vi "getImage.vi"(4 "Streeam":bool, 5 "imageError IN":errorcluster, 6 "Image IN":T1, 7 "errorCamera IN":errorcluster, 8 "hCamera IN":u32) -> (0 "errorImage OUT":errorcluster, 1 "Image OUT":T1, 2 "errorCamera OUT":errorcluster, 3 "hCamera OUT":u32)   [LabVIEW 2010]
uses:
  <vilib>/vision/Image Controls.llb/IMAQ Image.ctl
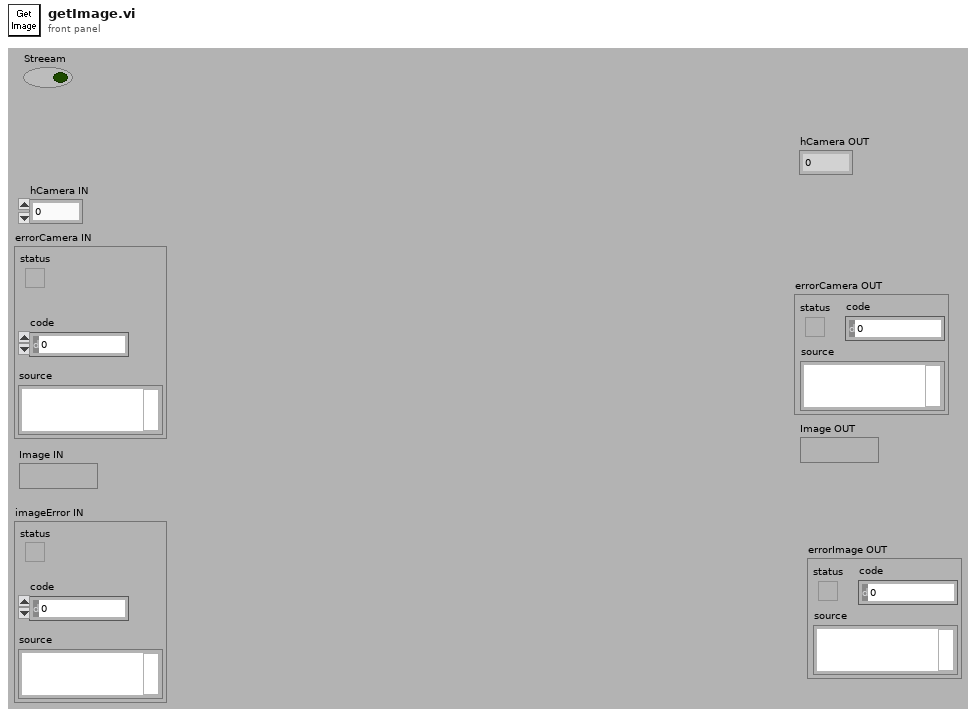
[diagram p1: front panel]
types:
  T1 = typedef "IMAQ Image.ctl" = refnum<image>
  T2 = enum32{"Map Pixel Pointer", "Unmap Pixel Pointer", "Get Pixels Infos"}
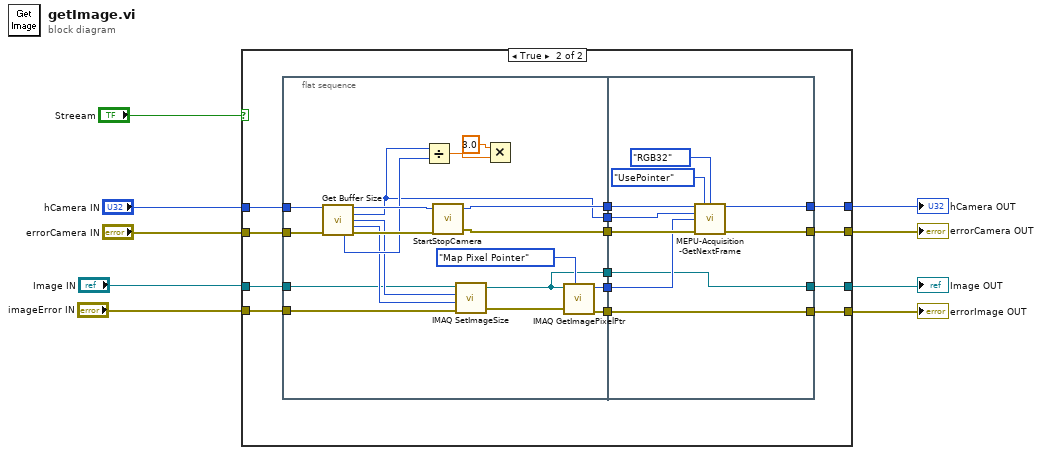
[diagram p0: block diagram]
diagram:
  n1 = case shown="True" "Streeam" {
    tunnel: "hCamera IN" -> [w13 w22]
    tunnel: "errorCamera IN" -> [w12 w21]
    tunnel: "Image IN" -> [w11 w20]
    tunnel: "imageError IN" -> [w10 w19]
    tunnel: [w11 w18] -> w4
    tunnel: [w10 w17] -> w3
    tunnel: [w12 w16] -> w2
    tunnel: [w13 w15] -> w1
    frame False {
    }
    frame True {
      n2 = flat-sequence {
        tunnel: [w44] -> w27
        tunnel: [w43] -> w26
        tunnel: w20 -> [w37]
        tunnel: w19 -> [w36]
        tunnel: w22 -> [w35]
        tunnel: w21 -> [w34]
        tunnel: [w31] -> w25
        tunnel: [w30] -> w24
        tunnel: [w29] -> w23
        tunnel: [w28] -> w14
        tunnel: w27 -> [w56]
        tunnel: w26 -> [w55]
        tunnel: w25 -> [w51]
        tunnel: w24 -> [w48]
        tunnel: w23 -> [w49]
        tunnel: [w50] -> w15
        tunnel: [w49] -> w18
        tunnel: [w48] -> w17
        tunnel: [w47] -> w16
        tunnel: w14 -> [w54]
        frame #0 {
          n3 = call "Get Buffer Size.vi"("phCamera IN"=w35, "Error IN"=w34) -> ("phCamera OUT"=w46:u32, "uBufferSize OUT"=w28:u32, "uWidth OUT"=w39:u32, "uHeight OUT"=w38:u32, "uBytesPerPixel OUT"=w40:u32, "Error OUT"=w45:errorcluster)  [unwired: 8 out]
          n4 = Divide(x=w28, y=w40) -> (x/y=w42:dbl)
          n5 = call "StartStopCamera.vi"("Error IN"=w45, "hCamera IN"=w46) -> ("Error OUT"=w43:errorcluster, "hCamera OUT"=w44:u32)  [unwired: 2 in]
          n6 = call "IMAQ SetImageSize"("error in (no error)"=w36, "Y Resolution"=w38, "X Resolution"=w39, "Image"=w37) -> ("error out"=w33:errorcluster, "Image Out"=w29:T1)  [unwired: 1 in]
          n7 = Multiply(x=3.0, y=w42) -> ()  [unwired: 1 out]
          n8 = call "IMAQ GetImagePixelPtr"("Function"=T2."Map Pixel Pointer", "error in (no error)"=w33, "Image"=w29) -> ("error out"=w30:errorcluster, "Pixel Pointer out"=w31:u64)  [unwired: 3 in, 4 out]
        }
        frame #1 {
          n9 = call <vilib>:"MEPU-Acquisition-GetNextFrame.vi"("hCamera IN"=w56, "Mode IN"=enum16{"UseArray", "UsePointer"}."UsePointer", "OutputMode IN"=enum16{"Default", "RGB24", "RGB32"}."RGB32", "uBufferSize IN"=w54, "pPixel IN"=w51, "Error IN"=w55) -> ("hCamera OUT"=w50:u32, "Error OUT"=w47:errorcluster)  [unwired: 5 in, 3 out]
        }
      }
    }
  }
  "Image OUT" <- w4
  "errorImage OUT" <- w3
  "errorCamera OUT" <- w2
  "hCamera OUT" <- w1
